vi "Exercise5.vi"() -> ()   [LabVIEW 2019]
panel:
  out "Time Stamp":timestamp
  out "time string":string
  out "date string":string
  out "x+1":dbl
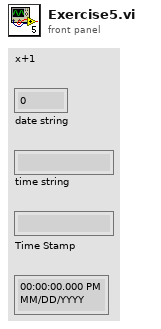
[diagram p1: front panel]
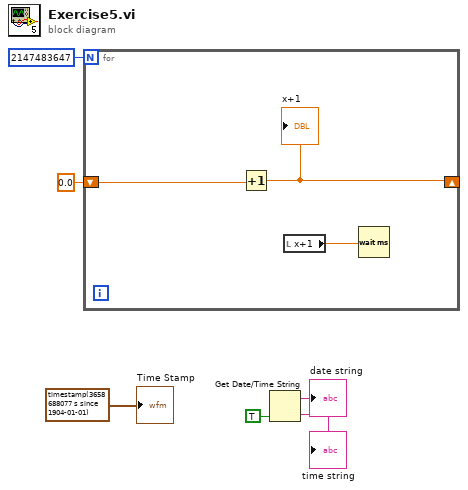
[diagram p0: block diagram]
diagram:
  n1 = for {
    N: 2147483647 -> [_]
    shift-right: [w9] -> _
    shift-left: 0.0 -> [w8]
    n2 = Increment(x=w8) -> (x+1=w9:dbl)
    "x+1" <- w9
    n3 = local read "x+1"() -> (w7:dbl)
    n4 = Wait (ms)(milliseconds to wait=w7) -> ()  [unwired: 1 out]
  }
  n5 = Get Date/Time String(want seconds? (F)=TRUE) -> (date string=→"date string":string, time string=→"time string":string)  [unwired: 2 in]
  "Time Stamp" <- timestamp(3658688077.163152 s since 1904-01-01)
